vi "Actor Core.vi"(8 "error in":errorcluster, 11 "Cobra RT in":refnum<class "Cobra RT.lvclass">) -> (0 "error out":errorcluster, 3 "Actor out":refnum<class "Actor.lvclass">)   [LabVIEW 2019, in "Cobra RT.lvlib" / "Cobra RT.lvclass"]
doc: "(<B>Filename</B>: Actor Framework.lvlib:Actor.lvclass:Actor Core.vi)\n\nReceives messages to the actor, reacts to them, and initiates any error handling that may shut the actor down.\n\nDescendant classes may override this VI to append parallel tasks for the actor to complete while it handles messages. Overrides use the Call Parent Method node."
uses:
  Cobra RT.lvclass
  C:/Program Files (x86)/National Instruments/LabVIEW 2019/vi.lib/MGI/Panel Manager/Panel Actor/Panel Actor/Panel Actor.lvclass
  <vilib>/ActorFramework/Actor/Actor.lvclass
  Cobra RT.lvclass/Cobra RT.ctl
  Test/Test Messages/NEA_Get Data Msg/NEA_Get Data Msg.lvclass/NEA_Get Data Msg.ctl
  <vilib>/ActorFramework/Message Enqueuer/Message Enqueuer.lvclass/Message Enqueuer.ctl
  <vilib>/ActorFramework/Message Enqueuer/Enqueue.vi
  Test/Test Messages/NEA_Get Data Msg/NEA_Get Data Msg.lvclass
  C:/Program Files (x86)/National Instruments/LabVIEW 2019/vi.lib/ActorFramework/Message/Message.lvclass
  <vilib>/ActorFramework/Stop Msg/Stop Msg.lvclass
  <vilib>/ActorFramework/Message Priority Queue/Priority Enqueue.vi
  <vilib>/MGI/Panel Manager/Panel Actor/Panel Actor/Panel Actor.lvclass
panel:
  in  "Data":T1={"M2 Dataset"={"Read Temp"=273.15, "Feedback"=1, "Set Temp"=273.15}, "M1 Dataset"={"Read Temp"=273.15, "Feedback"=1, "Set Temp"=273.15}, "Comp"=FALSE} {"M1 Dataset"."Set Temp" format="%.1f"; "M1 Dataset"."Feedback" items=["Evap Temp", "Case Temp", "Intec Temp", "TSD  Temp", "Autotune", "Extra"]; "M1 Dataset"."Read Temp" format="%.1f"; "M2 Dataset"."Set Temp" format="%.1f"; "M2 Dataset"."Feedback" items=["Evap Temp", "Case Temp", "Intec Temp", "TSD  Temp", "Autotune", "Extra"]; "M2 Dataset"."Read Temp" format="%.1f"}
  out "Setpoint":dbl=100.0
  out "Connected":bool
  # "degC"
  # "degC"
  # "degC"
  # "degC"
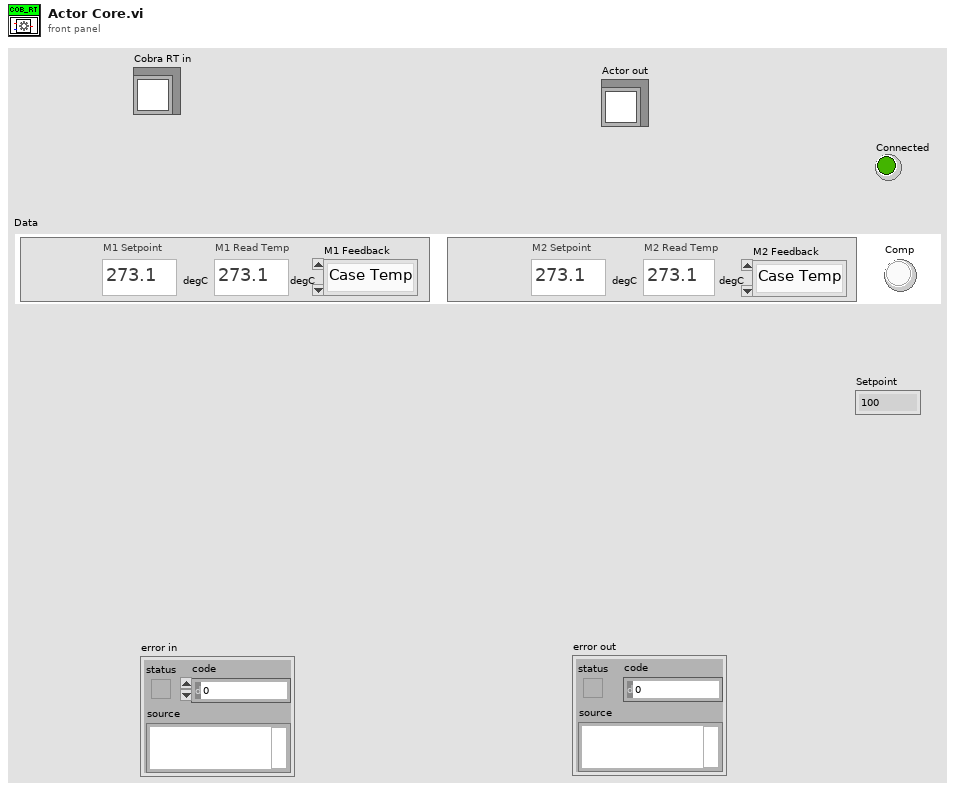
[diagram p1: front panel]
types:
  T1 = cluster{"M2 Dataset":cluster{"Read Temp":dbl, "Feedback":u8, "Set Temp":dbl}, "M1 Dataset":cluster{"Read Temp":dbl, "Feedback":u8, "Set Temp":dbl}, "Comp":bool}
  T2 = enum32{"Invalid", "Standard", "Closed", "Hidden", "Minimized", "Maximized"}
  T3 = cluster{"Connected":refnum<user-event>, "Setpoint":refnum<user-event>}
  T4 = cluster{"Event Registration Refnum":refnum<event-registration>, "Pnl Actor":refnum<event-registration>}
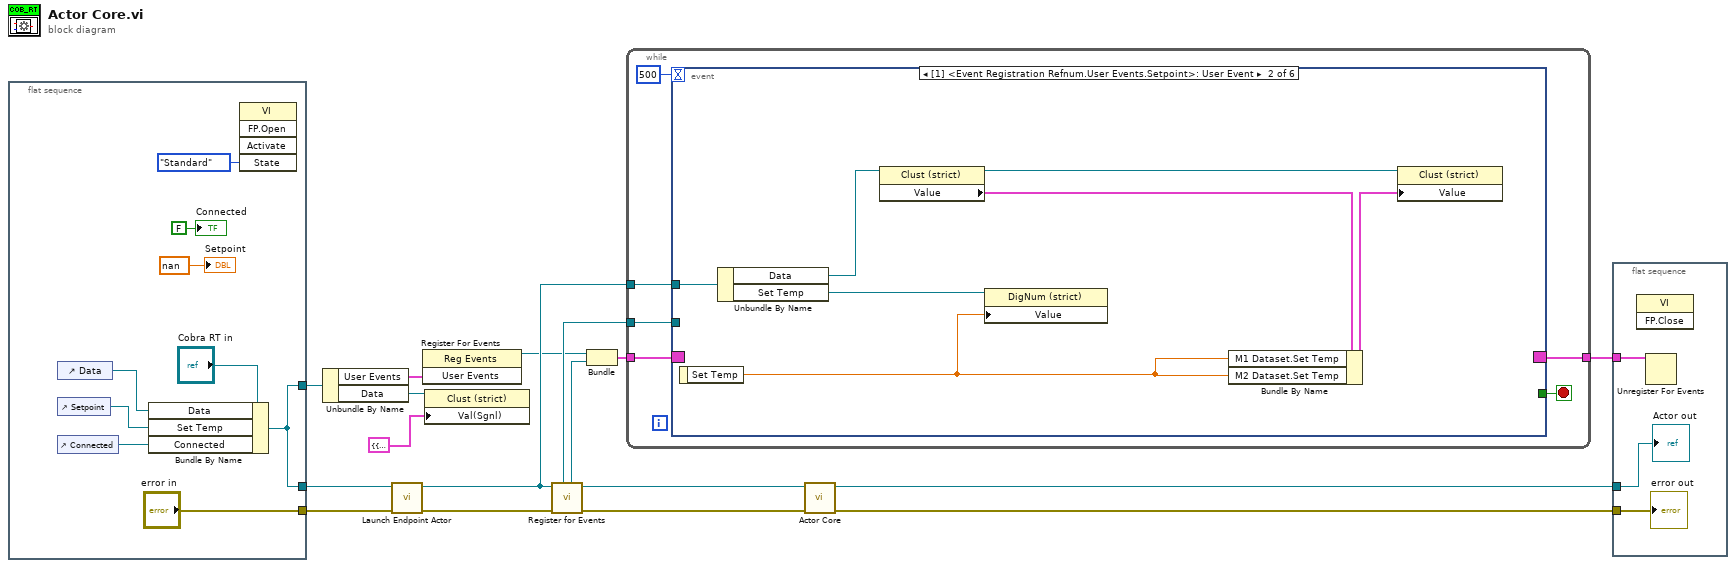
[diagram p0: block diagram]
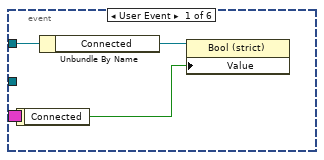
[diagram p2: hidden frame]
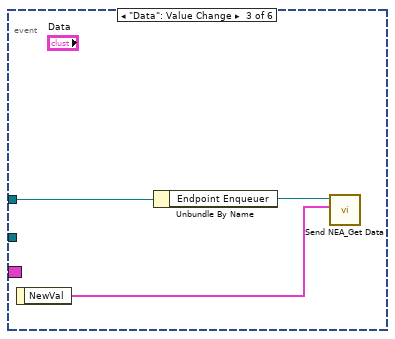
[diagram p3: hidden frame]
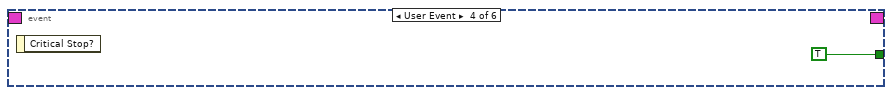
[diagram p4: hidden frame]
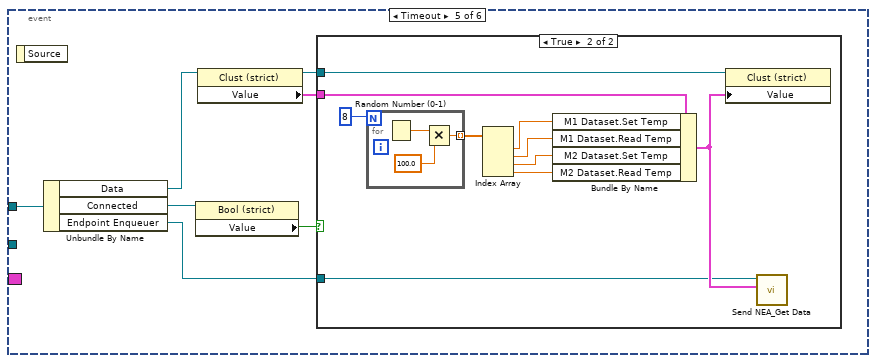
[diagram p5: hidden frame]
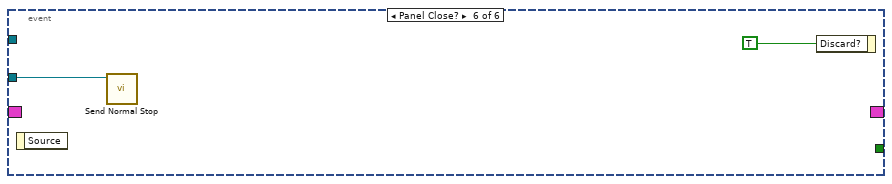
[diagram p7: hidden frame]
diagram:
  n1 = flat-sequence {
    tunnel: [w22] -> w14
    tunnel: ["error in"] -> w13
    tunnel: [w22] -> w11
    frame #0 {
      n2 = control-ref of="Data"() -> (w18:refnum<vi>)
      n3 = control-ref of="Setpoint"() -> (w19:refnum<vi>)
      n4 = control-ref of="Connected"() -> (w23:refnum<vi>)
      n5 = Bundle By Name(cluster="Cobra RT in", "Data"=w18, "Set Temp"=w19, "Connected"=w23) -> (w22:refnum<class "Cobra RT.lvclass">)
      n6 = invoke class="VI" method="FP.Open"("State"=T2."Standard") -> ()  [unwired: 4 in, 5 out]
      "Setpoint" <- nan
      "Connected" <- FALSE ("Connected")
    }
  }
  n7 = Unbundle By Name(w11) -> ("User Events"=w15:T3, "Data"=w3:refnum<vi>)
  n8 = call "Launch Endpoint Actor.vi"("error in (no error)"=w13, "Cobra RT in"=w14) -> ("error out"=w2:errorcluster, "Cobra RT out"=w10:refnum<class "Cobra RT.lvclass">)  [unwired: 8 in]
  n9 = register-events(w15) -> (reference out=w6:refnum<event-registration>)  [unwired: 2 in, 1 out]
  n10 = property class="Clust (strict)"(reference=w3, "Val(Sgnl)"=T1 {"M2 Dataset"={"Read Temp"=273.15, "Feedback"=1, "Set Temp"=273.15}, "M1 Dataset"={"Read Temp"=273.15, "Feedback"=1, "Set Temp"=273.15}, "Comp"=FALSE} ("Data")) -> ()  [unwired: 1 in, 2 out]
  n11 = call <vilib>:"Register for Events.vi"("Error In"=w2, "Panel Actor in"=w10) -> ("Error Out"=w9:errorcluster, "Panel Actor out"=w8:refnum<class "Cobra RT.lvclass">, "Pnl Actor"=w5:refnum<event-registration>, "Self Enqueuer"=w7:refnum<class "Message Enqueuer.lvclass">)  [unwired: 6 in]
  n12 = Bundle("Event Registration Refnum"=w6, "Pnl Actor"=w5) -> (w4:T4)  [unwired: 1 in]
  n13 = while {
    tunnel: w4 -> [w32]
    tunnel: [w30] -> w12
    tunnel: w7 -> [w29]
    tunnel: w10 -> [w28]
    stop <- w31 stop-if-true
    n14 = event shown="[1] <Event Registration Refnum.User Events.Setpoint>: User Event" {
      selector: w32 -> [_ _ _ _ _ _]
      dyn-events: [_ _ _ _ _ _] -> w30
      timeout: 500 -> [_ _ _ _ _ _]
      tunnel: [_ _ _ TRUE _ _] -> w31
      tunnel: w29 -> [_ _ _ _ _ w67]
      tunnel: w28 -> [w35 w42 w45 _ w53 _]
      event User Event {
        n15 = event-data() -> ("Connected"=w33:bool)  [unwired: 1 in]
        n16 = Unbundle By Name(w35) -> ("Connected"=w34:refnum<vi>)
        n17 = property class="Bool (strict)"(reference=w34, "Value"=w33) -> ()  [unwired: 1 in, 2 out]
      }
      event User Event {
        n18 = event-data() -> ("Set Temp"=w36:dbl)  [unwired: 1 in]
        n19 = Unbundle By Name(w42) -> ("Data"=w40:refnum<vi>, "Set Temp"=w41:refnum<vi>)
        n20 = property class="Clust (strict)"(reference=w40) -> (reference out=w38:refnum<vi>, "Value"=w39:T1)  [unwired: 1 in, 1 out]
        n21 = property class="DigNum (strict)"(reference=w41, "Value"=w36) -> ()  [unwired: 1 in, 2 out]
        n22 = Bundle By Name(cluster=w39, "M1 Dataset.Set Temp"=w36, "M2 Dataset.Set Temp"=w36) -> (w37:T1)
        n23 = property class="Clust (strict)"(reference=w38, "Value"=w37) -> ()  [unwired: 1 in, 2 out]
      }
      event "Data": Value Change {
        n24 = event-data() -> ("NewVal"=w43:T1)  [unwired: 1 in]
        n25 = Unbundle By Name(w45) -> ("Endpoint Enqueuer"=w44:refnum<class "Message Enqueuer.lvclass">)
        n26 = call "Send NEA_Get Data.vi"("Data"=w43, "Message Enqueuer"=w44) -> ()  [unwired: 8 in, 2 out]
      }
      event User Event {
        n27 = event-data() -> ()  [unwired: 1 in, 1 out]
      }
      event Timeout {
        n28 = event-data() -> ()  [unwired: 1 in, 1 out]
        n29 = Unbundle By Name(w53) -> ("Data"=w50:refnum<vi>, "Connected"=w52:refnum<vi>, "Endpoint Enqueuer"=w47:refnum<class "Message Enqueuer.lvclass">)
        n30 = property class="Bool (strict)"(reference=w52) -> ("Value"=w51:bool)  [unwired: 1 in, 2 out]
        n31 = property class="Clust (strict)"(reference=w50) -> (reference out=w48:refnum<vi>, "Value"=w49:T1)  [unwired: 1 in, 1 out]
        n32 = case shown="True" w51 {
          tunnel: w49 -> [_ w63]
          tunnel: w48 -> [_ w62]
          tunnel: w47 -> [_ w56]
          frame False {
          }
          frame True {
            n33 = for {
              N: 8 -> [_]
              tunnel: [w64] -> w60 mode=indexing
              n34 = Random Number (0-1)() -> (number: 0 to 1=w66:dbl)
              n35 = Multiply(x=w66, y=100.0) -> (x*y=w64:dbl)
            }
            n36 = Index Array(array=w60) -> (element #1=w59:dbl, element #2=w58:dbl, element #3=w55:dbl, element #4=w54:dbl)  [unwired: 4 in]
            n37 = Bundle By Name(cluster=w63, "M1 Dataset.Set Temp"=w59, "M1 Dataset.Read Temp"=w58, "M2 Dataset.Set Temp"=w55, "M2 Dataset.Read Temp"=w54) -> (w57:T1)
            n38 = property class="Clust (strict)"(reference=w62, "Value"=w57) -> ()  [unwired: 1 in, 2 out]
            n39 = call "Send NEA_Get Data.vi"("Data"=w57, "Message Enqueuer"=w56) -> ()  [unwired: 8 in, 2 out]
          }
        }
      }
      event Panel Close? {
        n40 = event-data() -> ()  [unwired: 1 in, 1 out]
        n41 = call <vilib>:"Send Normal Stop.vi"("Message Enqueuer"=w67) -> ()  [unwired: 10 in, 1 out]
        n42 = event-data("Discard?"=TRUE) -> ()  [unwired: 1 in, 1 out]
      }
    }
  }
  n43 = call-parent "Actor Core.vi"("error in"=w9, "Panel Actor in"=w8) -> ("error out"=w17:errorcluster, "Actor out"=w16:refnum<class "Actor.lvclass">)  [unwired: 8 in]
  n44 = flat-sequence {
    tunnel: w17 -> [w71]
    tunnel: w16 -> [w70]
    tunnel: w12 -> [w69]
    frame #0 {
      n45 = invoke class="VI" method="FP.Close"() -> ()  [unwired: 3 in, 3 out]
      n46 = Unregister For Events(event registration refnum=w69) -> ()  [unwired: 1 in, 1 out]
      "error out" <- w71
      "Actor out" <- w70
    }
  }
